vi "Helper-Cluster.vi"() -> ()   [LabVIEW 2016]
uses:
  Typedef/OperationControl.ctl
  Typedef/NumberControl.ctl
  Typedef/BooleanControl.ctl
panel:
  out "Boolean":T1
  in  "Number":T2
  in  "Operation":T3
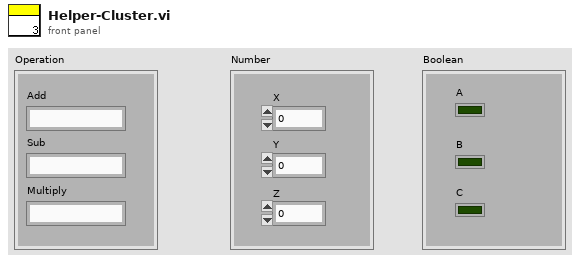
[diagram p1: front panel]
types:
  T1 = typedef "BooleanControl.ctl" = cluster{"A":bool, "B":bool, "C":bool}
  T2 = typedef "NumberControl.ctl" = cluster{"X":dbl, "Y":dbl, "Z":dbl}
  T3 = typedef "OperationControl.ctl" = cluster{"Add":string, "Sub":string, "Multiply":string}
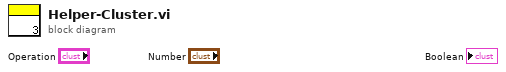
[diagram p0: block diagram]
diagram:
